vi "ShutdownServerCon.vi"(5 "error in":T1) -> (19 "error out":T1)   [LabVIEW 2016]
doc: "This VI closes the connection to the server and therefore presents the last VI concerning the ASC500 in an application."
uses:
  Controls/Error_Out.ctl
  Files_ASC500/DLL/ASC500_RemoteControlV27.dll
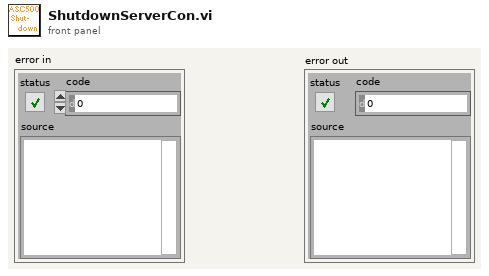
[diagram p1: front panel]
types:
  T1 = typedef "Error_Out.ctl" = errorcluster
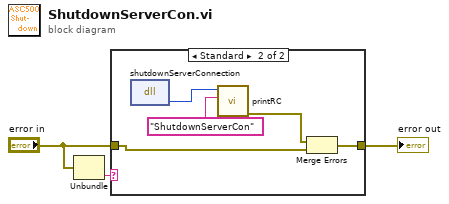
[diagram p0: block diagram]
diagram:
  n1 = Unbundle("error in") -> ("source"=w3:string)  [unwired: 2 out]
  n2 = case shown="Standard" w3 {
    tunnel: [w4 w5] -> w2
    tunnel: "error in" -> [w4 w7]
    frame "Init" {
    }
    frame Default {
      n3 = dll-call lib="G:/SCMOperations/Share/ELE/Produkt Information/ASC500/04 Remote Control/02 development versions/2018Nov06/Files_ASC500/DLL/ASC500_RemoteControlV27.dll" fn="shutdownServerConnection"() -> ("return type"=w9:i32)  [unwired: 3 in, 2 out]
      n4 = call "printRC.vi"("additional information"="ShutdownServerCon", "RC"=w9) -> ("error out"=w6:T1)  [unwired: 9 in]
      n5 = Merge Errors(w6, w7) -> (w5:errorcluster)
    }
  }
  "error out" <- w2
